vi "Scan Setup.vi"(8 "error in (no error)":errorcluster, 11 "Analog Out Scan in":refnum<class "Analog Output Scan.lvclass">) -> (0 "error out":errorcluster, 3 "Analog Out Scan out":refnum<class "Analog Output Scan.lvclass">)   [LabVIEW 2023, in "Analog Output Scan.lvclass"]
doc: "Configure the Instrument based on the class member fields. This step comes after the user has closed the \"Scan Setup\" window and before the actual scan -- so instruments are configured with the user's specified settings."
uses:
  Analog Output Scan.lvclass
  Analog Output Scan.lvclass/Analog Output Scan.ctl
  <vilib>/DAQmx/create/channels.llb/DAQmx Create Channel (AO-Voltage-Basic).vi
  Scanner/Scanner.lvclass
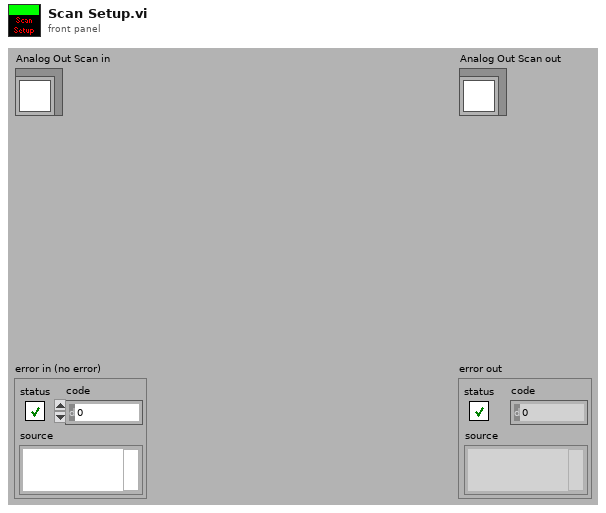
[diagram p1: front panel]
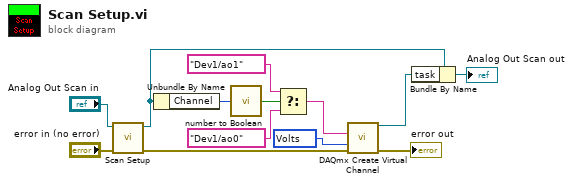
[diagram p0: block diagram]
diagram:
  w1 = 10348 items=["Volts"=10348, "From Custom Scale"=10065] ("units")
  n1 = call-parent "Scan Setup.vi"("error in (no error)"="error in (no error)", "Scanner in"="Analog Out Scan in") -> ("error out"=w3:errorcluster, "Scanner out"=w5:refnum<class "Analog Output Scan.lvclass">)  [unwired: 8 in]
  n2 = Unbundle By Name(w5) -> ("Channel"=w11:u8)
  n3 = call "number to Boolean.vi"("Numeric"=w11) -> ("Boolean"=w10:bool)
  n4 = Select(t=tag "Dev1/ao1" ("physical channels"), s=w10, f=tag "Dev1/ao0" ("physical channels")) -> (s? t:f=w7:tag)
  n5 = call-poly <vilib>:"DAQmx Create Virtual Channel.vi"("physical channels"=w7, "units"=w1, "error in"=w3) -> ("task out"=w6:refnum<k21>, "error out"=→"error out":errorcluster)  [unwired: 11 in]
  n6 = Bundle By Name(cluster=w5, "task"=w6) -> (→"Analog Out Scan out":refnum<class "Analog Output Scan.lvclass">)
